vi "util_gen_cmd_error.vi"(8 "error in (no error)":errorcluster, 10 "return_code":i32, 11 "standard_error":string) -> (0 "error out":errorcluster)   [LabVIEW 2015, in "lv-bin.lvlib" / "v1.lvlib"]
uses:
  v1.lvlib
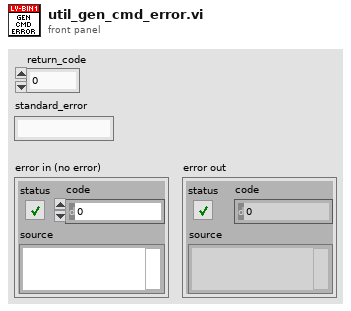
[diagram p1: front panel]
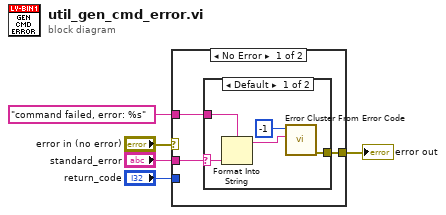
[diagram p0: block diagram]
diagram:
  n1 = case shown="No Error" "error in (no error)" {
    selector: "error in (no error)" -> [_ w14]
    tunnel: [w7 w14] -> w4
    tunnel: "standard_error" -> [w6 _]
    tunnel: "command failed, error: %s" ("format string") -> [w8 _]
    tunnel: "return_code" -> [_ _]
    frame No Error {
      n2 = case shown="Default" w6 {
        selector: w6 -> [w9 _]
        tunnel: w8 -> [w13 _]
        tunnel: [w12 _] -> w7
        frame Default {
          n3 = Format Into String(format string=w13, w9) -> (resulting string=w11:string)  [unwired: 2 in, 1 out]
          n4 = call <vilib>:"Error Cluster From Error Code.vi"("error message (\"\")"=w11, "error code (0)"=-1) -> ("error out"=w12:errorcluster)  [unwired: 7 in]
        }
        frame "" {
        }
      }
    }
    frame Error {
    }
  }
  "error out" <- w4
